vi "Intellirupter_basic.vi"() -> ()   [LabVIEW 2016]
uses:
  <vilib>/addons/Electrical Power/Protection/Definite Time Delay/subVIs/fpga_Time Delay Cfg.ctl
  <vilib>/FPGAPlugInAG/cRIO-9039 (Sync)/niLvFpga_Open_cRIO-9039 (Sync).vi
  <vilib>/rvi/interface/common/dynamic/niFpgaDynamicAddResources.vi
  <vilib>/Utility/error.llb/Error Cluster From Error Code.vi
  <vilib>/rvi/errors/niLvFpgaAdjustHostInterfaceError.vi
  <vilib>/FPGAPlugInAG/Dynamic/niLvFpga_Close_Dynamic.vi
  <vilib>/rvi/interface/nirviOpenFPGA/nirviOpenFPGA.xnode
  FPGA Bitfiles/IntelliRupter_calibrated.lvbitx
  <vilib>/rvi/interface/nirviReadWriteControl/nirviReadWriteControl.xnode
  <vilib>/rvi/interface/nirviCloseFPGA/nirviCloseFPGA.xnode
  <vilib>/rvi/interface/Simulation/niFpgaSimulationCallBeginRW.vi
  NiFpgaLv.dll
  <vilib>/addons/Electrical Power/Protection/NI_EP_Protection_FPGA.lvlib
panel:
  out "x-y":u32=48
  in  "Recloser Settings":T1={"Magnitude Minimum"=0.1, "Magnitude difference level"=0.005, "Frequency difference level"=0.5, "Phase difference level"=10.0}
  out "Trip Relay8":bool
  out "Trip Relay7":bool
  out "Trip Relay6":bool
  out "Trip Relay5":bool
  out "Trip Relay4":bool
  out "Trip Relay3":bool=TRUE
  out "Trip Relay2":bool
  out "Trip Relay1":bool
  out "MGCC_to_relay":bool[](array[boolean])=[TRUE, TRUE, FALSE, TRUE, TRUE, TRUE, TRUE, TRUE]
  out "Waveform Chart":dbl(graph)=-0.6613750457763672
  in  "Count(ticks)":u32=10000
  in  "RMS minimum\nvalues":T2={"VRMS values"=[0.5, 0.5, 0.5], "IRMS values"=[0.1, 0.1, 0.1]}
  out "error out":errorcluster
  out "Relay_toMGCC":bool[](array[boolean])=[TRUE, TRUE, FALSE, TRUE, TRUE, TRUE, TRUE, TRUE]
  in  "Manual trip Relay8":bool
  in  "Reclose Relay8?":bool=TRUE
  out "R8 Data for\ncommunication":dbl[](array[numeric])=[1.0, 0.9772472927114874, 0.9778624121532871, 61.827518463134766, 61.82509231567383, -3.8680694103240967, 0.13812482357025146, 0.006883656140416861, 0.0, 0.0]
  in  "Manual trip Relay7":bool
  in  "Reclose Relay7?":bool=TRUE
  out "R7 Data for\ncommunication":dbl[](array[numeric])=[1.0, 0.9791859731446678, 0.9754579902644022, 61.867767333984375, 61.880252838134766, -0.6613750457763672, -0.12970688939094543, -0.04306116700172424, 0.0, 0.0]
  in  "Manual trip Relay6":bool
  in  "Reclose Relay6?":bool=TRUE
  out "R6 Data for\ncommunication":dbl[](array[numeric])=[1.0, 0.9788151236253823, 0.9740843633835886, 61.9020881652832, 61.9046630859375, -2.975890874862671, 0.1713959127664566, 0.006507526151835918, 0.0, 0.0]
  in  "Manual trip Relay5":bool
  in  "Reclose Relay5?":bool=TRUE
  out "R5 Data for\ncommunication":dbl[](array[numeric])=[1.0, 0.9783700429887375, 0.9755752232502363, 61.90061569213867, 61.932212829589844, -2.8843889236450195, 0.1442330777645111, 0.0923943892121315, 0.0, 0.0]
  in  "Manual trip Relay4":bool
  in  "Reclose Relay4?":bool=TRUE
  out "R4 Data for\ncommunication":dbl[](array[numeric])=[1.0, 0.9780153533539752, 0.9771056813373646, 61.89913558959961, 61.91067123413086, 0.8295685648918152, 0.14155393838882446, 0.10946153849363327, 0.0, 0.0]
  in  "Manual trip Relay3":bool
  in  "Reclose Relay3?":bool
  out "R3 Data for\ncommunication":dbl[](array[numeric])=[0.0, 0.9772597508136373, 0.0028412240837732733, 61.94487380981445, 60.0, 87.80017852783203, 0.0009702712413854897, -0.00019450465333648026, 0.0, 0.0]
  in  "Manual trip Relay2":bool
  in  "Reclose Relay2?":bool=TRUE
  out "R2 Data for\ncommunication":dbl[](array[numeric])=[1.0, 0.9799129313520322, 0.9783522289749266, 61.984336853027344, 61.987144470214844, 4.425566673278809, 0.5318686962127686, 0.09335238486528397, 0.0, 0.0028076171875]
  out "R1 Data for\ncommunication":dbl[](array[numeric])=[1.0, 0.9830398860987186, 0.9848198490696459, 62.0186653137207, 62.001502990722656, 3.7592506408691406, 0.7891018986701965, 0.08714056760072708, 0.0, -0.017162322998046875]
  in  "Relay8":bool=TRUE
  in  "Relay7":bool=TRUE
  in  "Relay6":bool=TRUE
  in  "Relay5":bool=TRUE
  in  "Relay4":bool=TRUE
  in  "Relay3":bool
  in  "Relay2":bool=TRUE
  in  "Reclose Relay1?":bool=TRUE
  out "half cycle (samples)":i32=96
  out "basic calc interval":u16=2074
  in  "stop":bool
  in  "Relay1":bool=TRUE
  in  "Manual trip Relay1":bool
  # "status\nmag_left\nmag_right\nfreq_left\nfreq_right\nang_diff\nact_power\nrea_power\n0\n0"
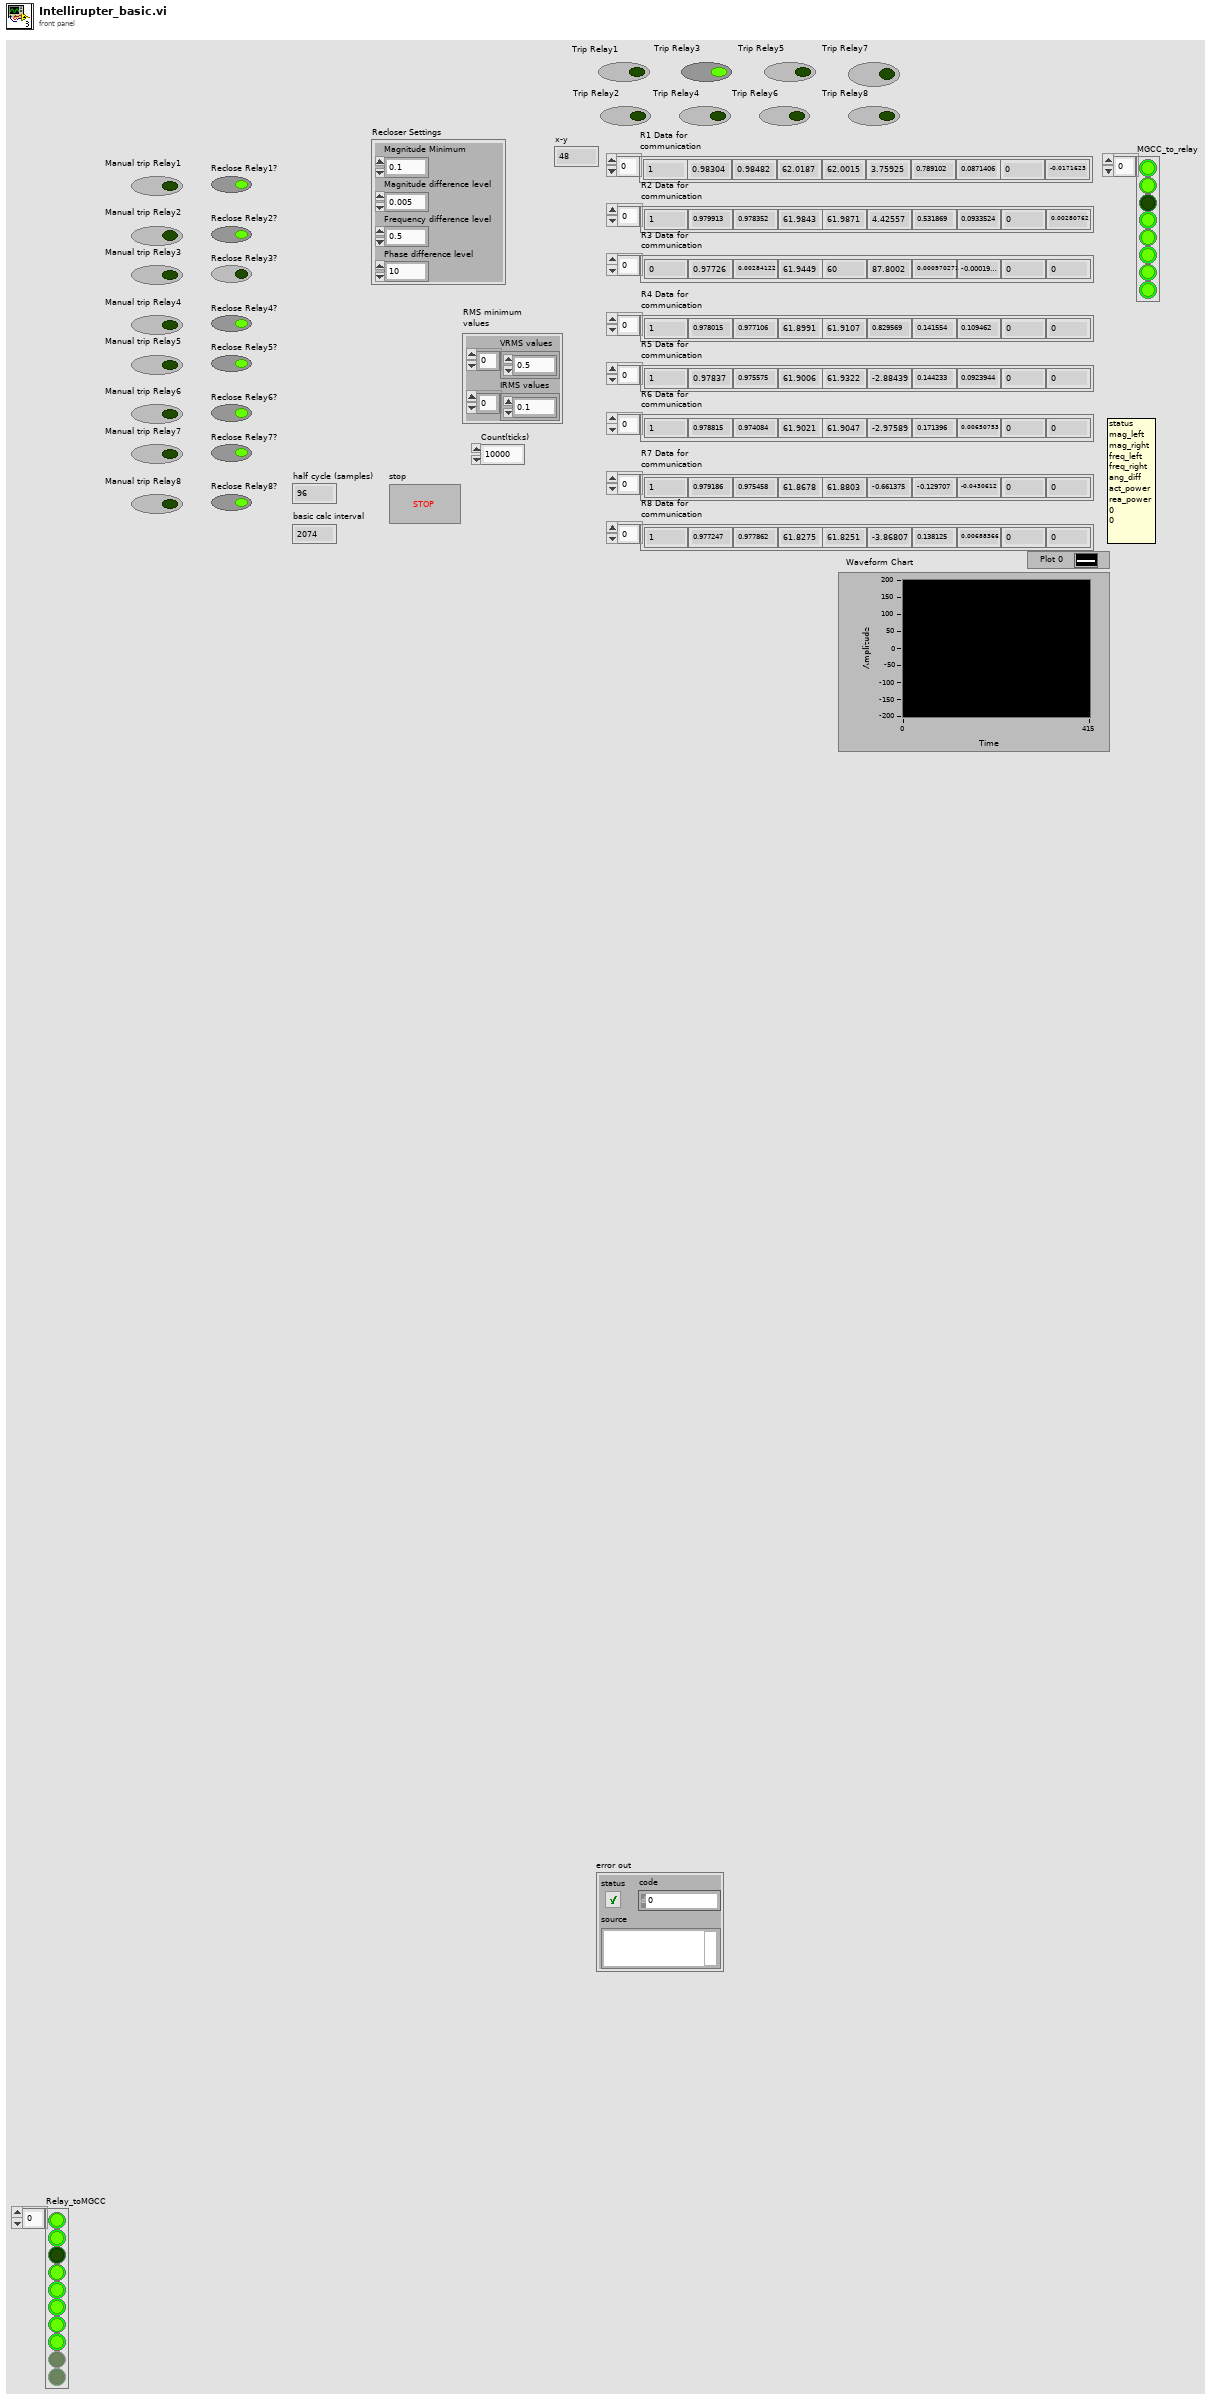
[diagram p1: front panel]
types:
  T1 = cluster{"Magnitude Minimum":dbl, "Magnitude difference level":dbl, "Frequency difference level":dbl, "Phase difference level":dbl}
  T2 = cluster{"VRMS values":dbl[], "IRMS values":dbl[]}
  T3 = cluster{fxp<+/-,53,11>[], fxp<+/-,53,11>[], fxp<+/-,53,11>[], fxp<+/-,53,11>[], fxp<+/-,53,11>[], fxp<+/-,53,11>[], fxp<+/-,53,11>[], fxp<+/-,53,11>[], fxp<+/-,53,11>[]}
  T4 = typedef "NI_EP_Protection_FPGA.lvlib/fpga_Time Delay Cfg.ctl" = cluster{"operate time [ms]":u32, "reset time [ms]":u32, "operate time compensation [ms]":u32}
  T5 = cluster{"UV Reset level":dbl, "Undervoltage \npick-up level":dbl, "OC Reset level":dbl, "Overcurrent\npick-up level":dbl, "time delay settings":T4}
  T6 = typedef "NI_EP_Protection_FPGA.lvlib/fpga_Timer Feedback Var.ctl" = cluster{"time elapsed":u32, "start time of trip counting":u32, "start time of reseting":u32}
  T7 = typedef "NI_EP_Protection_FPGA.lvlib/fpga_State.ctl" = enum16{"Idle", "Trip Counting", "Tripped", "Reset Counting"}
  T8 = cluster{bool, bool, "Boolean":bool, "timing values out":T6, "status out":T7, "trip signal out":bool}
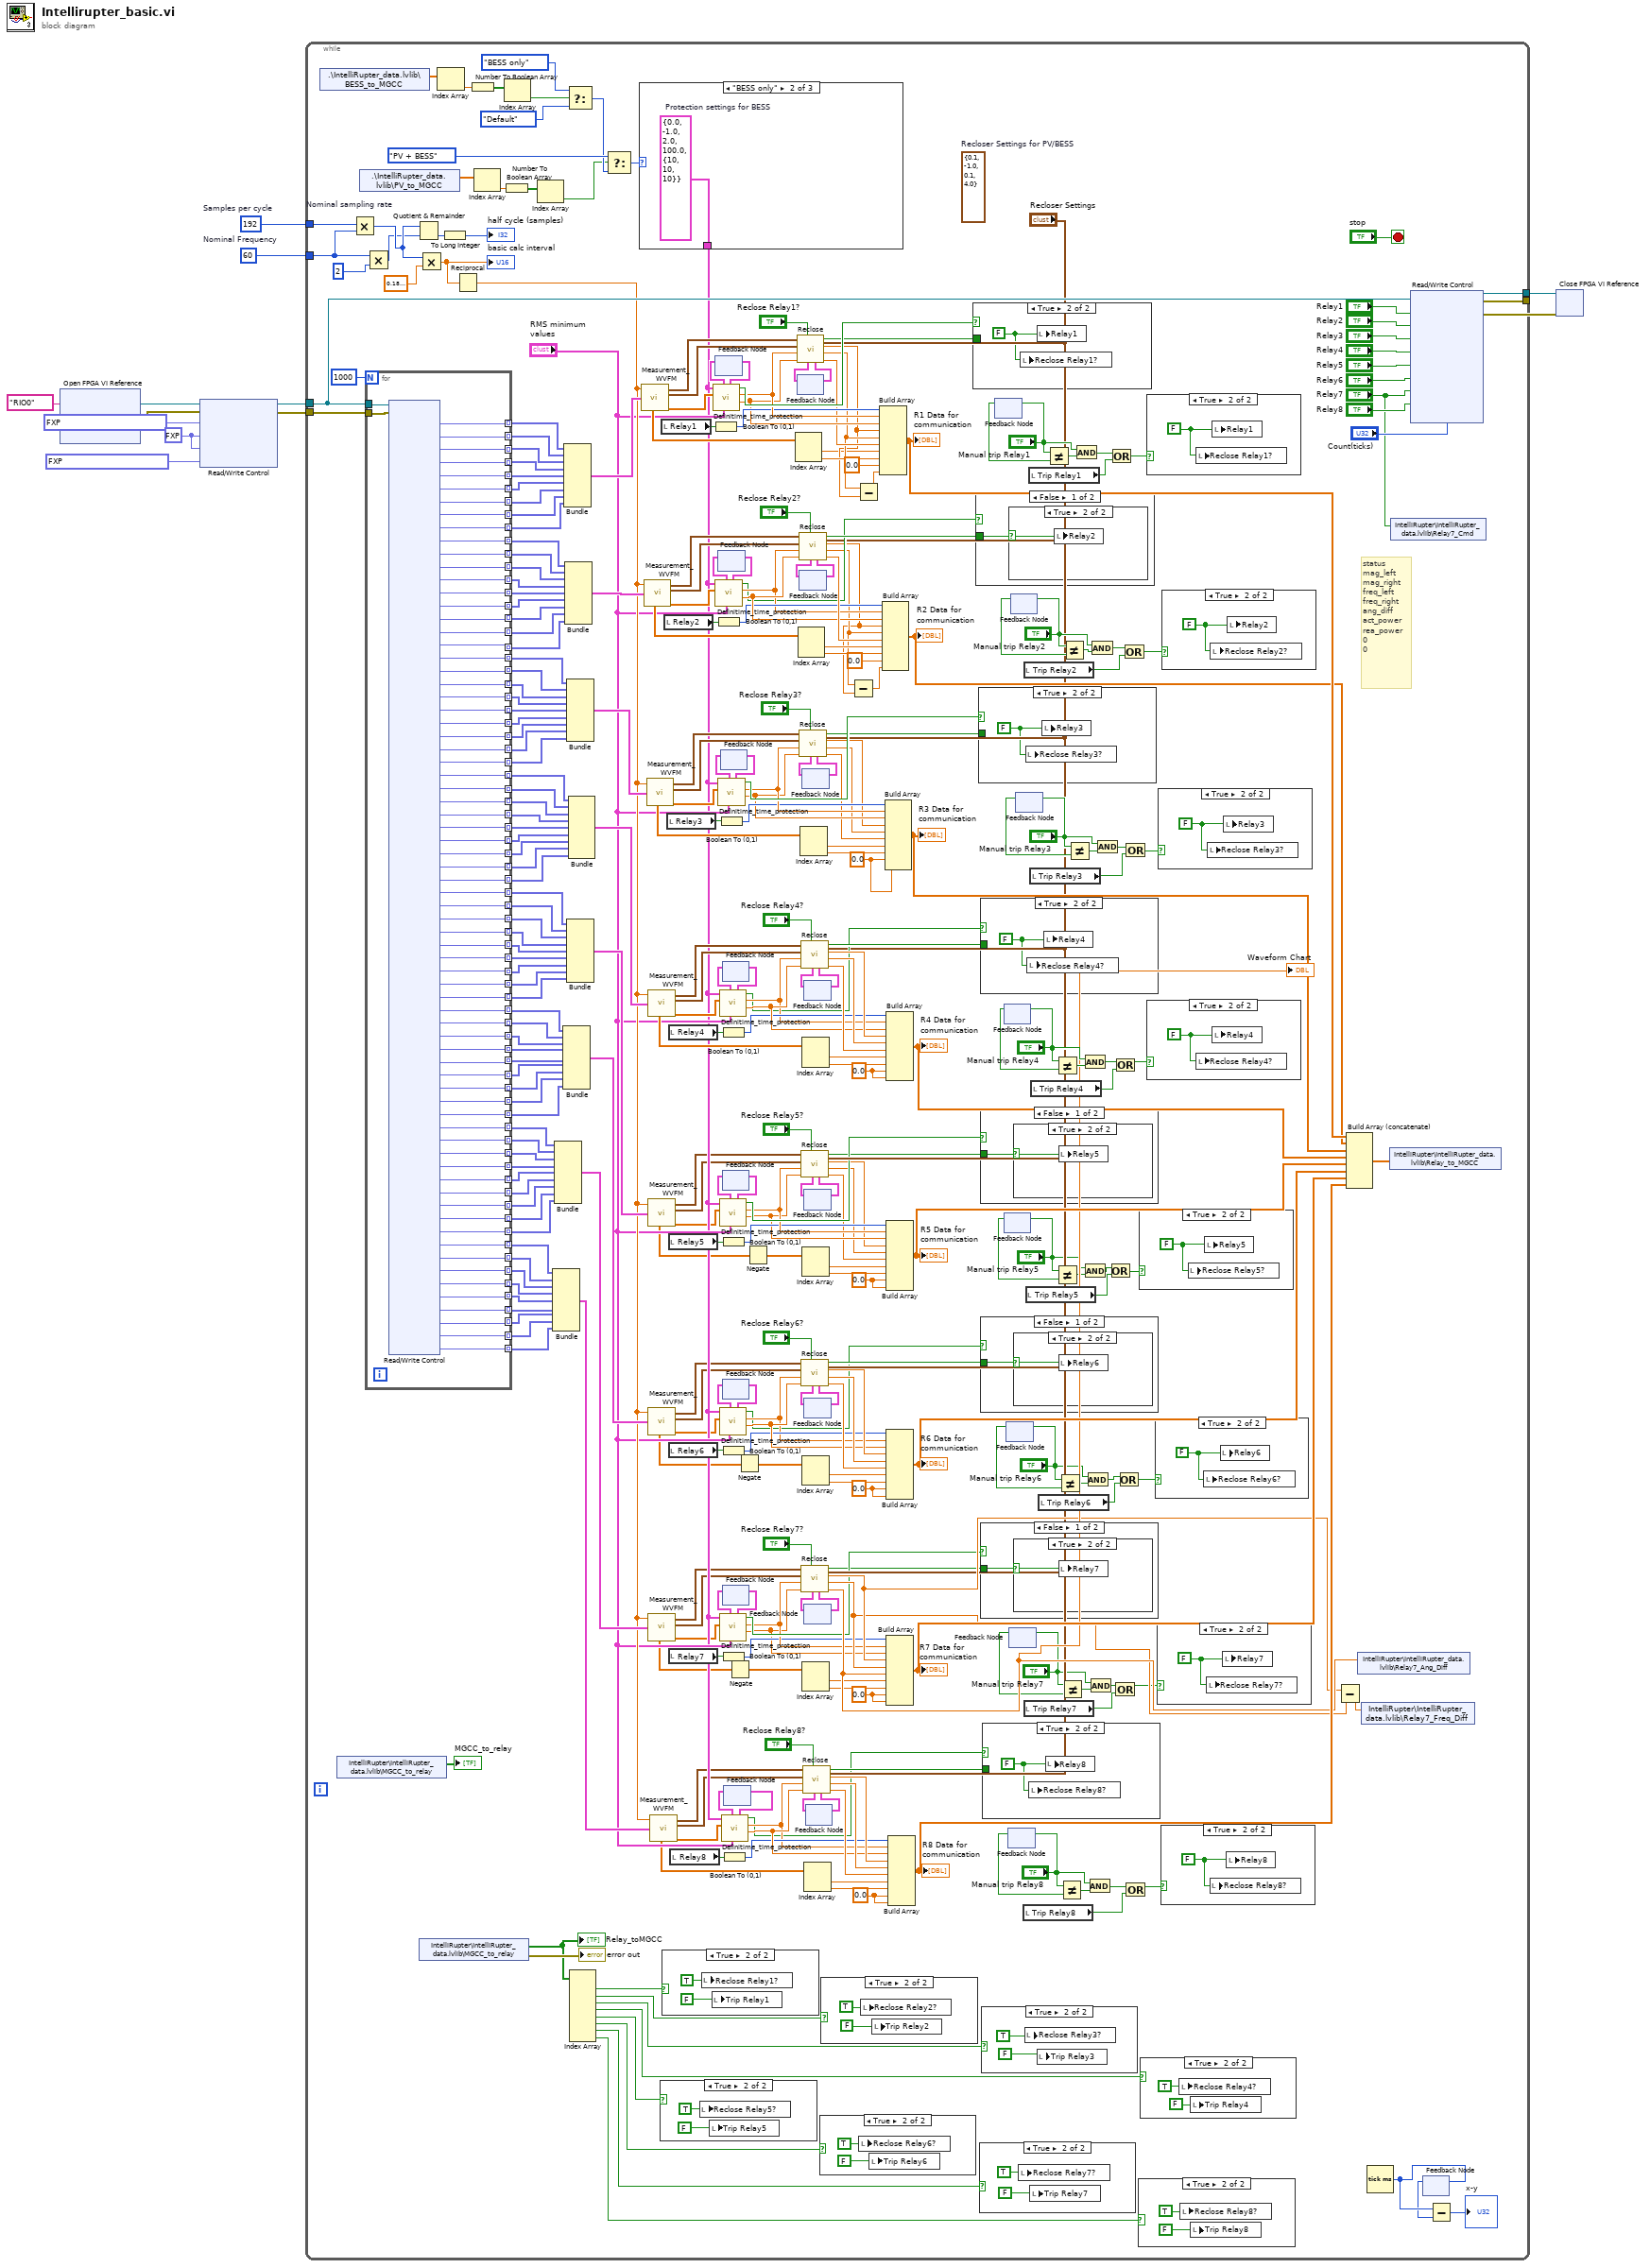
[diagram p0: block diagram]
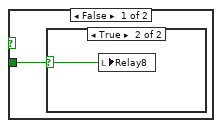
[diagram p2: hidden frame]
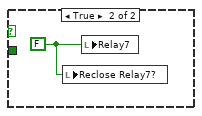
[diagram p6: hidden frame]
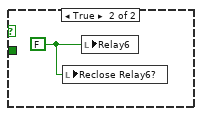
[diagram p9: hidden frame]
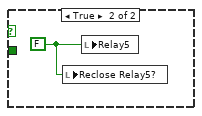
[diagram p12: hidden frame]
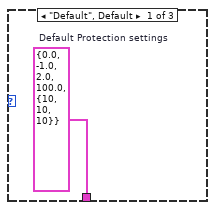
[diagram p14: hidden frame]
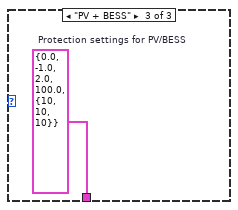
[diagram p15: hidden frame]
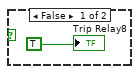
[diagram p16: hidden frame]
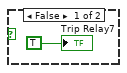
[diagram p17: hidden frame]
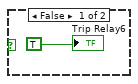
[diagram p18: hidden frame]
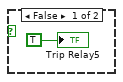
[diagram p19: hidden frame]
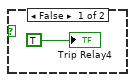
[diagram p20: hidden frame]
diagram:
  w2 = fxp<+/-,52,10> 0.0 ("I offset")
  w1 = 192  # Samples per cycle
  w10 = 60  # Nominal Frequency
  n1 = xnode "Open FPGA VI Reference"("resource name"=tag "RIO0") -> ("FPGA VI Reference Out"=w12:refnum<k20>, "error out"=w6:errorcluster)  [unwired: 1 in]
  n2 = xnode "Read/Write Control"("FPGA VI Reference In"=w12, "error in"=w6, "I scale factor"=fxp<+/-,26,5> 0.4850001335144043, "I offset"=w2, "V offset"=w2, "V scale factor"=fxp<+/-,26,5> 0.40000009536743164) -> ("FPGA VI Reference Out"=w7:refnum<k20>, "error out"=w5:errorcluster)
  n3 = while {
    tunnel: w7 -> [w363]
    tunnel: w10 -> [w371]
    tunnel: [w369] -> w9
    tunnel: [w368] -> w8
    tunnel: w5 -> [w362]
    tunnel: w1 -> [w176]
    stop <- "stop" stop-if-true
    w62 = 0.0 ("element")
    w63 = 0.0 ("element")
    w106 = 0.0 ("element")
    w107 = 0.0 ("element")
    (unwired) T1 {"Magnitude Minimum"=0.1, "Magnitude difference level"=-1.0, "Frequency difference level"=0.1, "Phase difference level"=4.0}  # Recloser Settings for PV/BESS
    w262 = 0.0 ("element")
    w272 = 0.0 ("element")
    # "status\nmag_left\nmag_right\nfreq_left\nfreq_right\nang_diff\nact_power\nrea_power\n0\n0"
    n4 = shared-variable ".\\IntelliRupter_data.lvlib\\BESS_to_MGCC"() -> (w134:dbl[])  [unwired: 1 in, 1 out]
    n5 = shared-variable "IntelliRupter\\IntelliRupter_data.lvlib\\MGCC_to_relay"() -> (→"MGCC_to_relay":bool[])  [unwired: 1 in, 1 out]
    n6 = Multiply "Nominal sampling rate"(x=w176, y=w371) -> (x*y=w377:i32)
    n7 = shared-variable ".\\IntelliRupter_data.lvlib\\PV_to_MGCC"() -> (w138:dbl[])  [unwired: 1 in, 1 out]
    n8 = Multiply(x=w371, y=2) -> (x*y=w373:i32)
    n9 = for {
      N: 1000 -> [_]
      tunnel: w363 -> [w507]
      tunnel: w362 -> [w506]
      tunnel: [w505] -> w360 mode=indexing
      tunnel: [w504] -> w359 mode=indexing
      tunnel: [w503] -> w358 mode=indexing
      tunnel: [w502] -> w357 mode=indexing
      tunnel: [w501] -> w356 mode=indexing
      tunnel: [w500] -> w355 mode=indexing
      tunnel: [w499] -> w354 mode=indexing
      tunnel: [w498] -> w353 mode=indexing
      tunnel: [w497] -> w352 mode=indexing
      tunnel: [w496] -> w326 mode=indexing
      tunnel: [w495] -> w325 mode=indexing
      tunnel: [w494] -> w324 mode=indexing
      tunnel: [w493] -> w323 mode=indexing
      tunnel: [w492] -> w322 mode=indexing
      tunnel: [w491] -> w321 mode=indexing
      tunnel: [w490] -> w320 mode=indexing
      tunnel: [w489] -> w319 mode=indexing
      tunnel: [w488] -> w318 mode=indexing
      tunnel: [w487] -> w271 mode=indexing
      tunnel: [w486] -> w270 mode=indexing
      tunnel: [w485] -> w269 mode=indexing
      tunnel: [w484] -> w268 mode=indexing
      tunnel: [w483] -> w267 mode=indexing
      tunnel: [w482] -> w266 mode=indexing
      tunnel: [w481] -> w265 mode=indexing
      tunnel: [w480] -> w264 mode=indexing
      tunnel: [w479] -> w263 mode=indexing
      tunnel: [w478] -> w237 mode=indexing
      tunnel: [w477] -> w236 mode=indexing
      tunnel: [w476] -> w235 mode=indexing
      tunnel: [w475] -> w234 mode=indexing
      tunnel: [w474] -> w233 mode=indexing
      tunnel: [w473] -> w232 mode=indexing
      tunnel: [w472] -> w231 mode=indexing
      tunnel: [w471] -> w230 mode=indexing
      tunnel: [w470] -> w229 mode=indexing
      tunnel: [w469] -> w228 mode=indexing
      tunnel: [w468] -> w227 mode=indexing
      tunnel: [w467] -> w226 mode=indexing
      tunnel: [w466] -> w225 mode=indexing
      tunnel: [w465] -> w224 mode=indexing
      tunnel: [w464] -> w223 mode=indexing
      tunnel: [w463] -> w222 mode=indexing
      tunnel: [w462] -> w221 mode=indexing
      tunnel: [w461] -> w220 mode=indexing
      tunnel: [w460] -> w218 mode=indexing
      tunnel: [w459] -> w217 mode=indexing
      tunnel: [w458] -> w216 mode=indexing
      tunnel: [w457] -> w215 mode=indexing
      tunnel: [w456] -> w214 mode=indexing
      tunnel: [w455] -> w213 mode=indexing
      tunnel: [w454] -> w212 mode=indexing
      tunnel: [w453] -> w211 mode=indexing
      tunnel: [w452] -> w210 mode=indexing
      tunnel: [w451] -> w208 mode=indexing
      tunnel: [w450] -> w207 mode=indexing
      tunnel: [w449] -> w206 mode=indexing
      tunnel: [w448] -> w205 mode=indexing
      tunnel: [w447] -> w204 mode=indexing
      tunnel: [w446] -> w203 mode=indexing
      tunnel: [w445] -> w202 mode=indexing
      tunnel: [w444] -> w201 mode=indexing
      tunnel: [w443] -> w200 mode=indexing
      tunnel: [w442] -> w198 mode=indexing
      tunnel: [w441] -> w197 mode=indexing
      tunnel: [w440] -> w196 mode=indexing
      tunnel: [w439] -> w195 mode=indexing
      tunnel: [w438] -> w194 mode=indexing
      tunnel: [w437] -> w193 mode=indexing
      tunnel: [w436] -> w192 mode=indexing
      tunnel: [w435] -> w191 mode=indexing
      tunnel: [w434] -> w190 mode=indexing
      n10 = xnode "Read/Write Control"("FPGA VI Reference In"=w507, "error in"=w506) -> ("V1L AB"=w505:fxp<+/-,53,11>, "V1L BC"=w504:fxp<+/-,53,11>, "V1L CA"=w503:fxp<+/-,53,11>, "V1R AB"=w502:fxp<+/-,53,11>, "V1R BC"=w501:fxp<+/-,53,11>, "V1R CA"=w500:fxp<+/-,53,11>, "I1 A"=w499:fxp<+/-,53,11>, "I1 B"=w498:fxp<+/-,53,11>, "I1 C"=w497:fxp<+/-,53,11>, "V2L AB"=w496:fxp<+/-,53,11>, "V2L BC"=w495:fxp<+/-,53,11>, "V2L CA"=w494:fxp<+/-,53,11>, "V2R AB"=w493:fxp<+/-,53,11>, "V2R BC"=w492:fxp<+/-,53,11>, "V2R CA"=w491:fxp<+/-,53,11>, "I2 A"=w490:fxp<+/-,53,11>, "I2 B"=w489:fxp<+/-,53,11>, "I2 C"=w488:fxp<+/-,53,11>, "V3L AB"=w487:fxp<+/-,53,11>, "V3L BC"=w486:fxp<+/-,53,11>, "V3L CA"=w485:fxp<+/-,53,11>, "V3R AB"=w484:fxp<+/-,53,11>, "V3R BC"=w483:fxp<+/-,53,11>, "V3R CA"=w482:fxp<+/-,53,11>, "I3 A"=w481:fxp<+/-,53,11>, "I3 B"=w480:fxp<+/-,53,11>, "I3 C"=w479:fxp<+/-,53,11>, "V4L AB"=w478:fxp<+/-,53,11>, "V4L BC"=w477:fxp<+/-,53,11>, "V4L CA"=w476:fxp<+/-,53,11>, "V4R AB"=w475:fxp<+/-,53,11>, "V4R BC"=w474:fxp<+/-,53,11>, "V4R CA"=w473:fxp<+/-,53,11>, "I4 A"=w472:fxp<+/-,53,11>, "I4 B"=w471:fxp<+/-,53,11>, "I4 C"=w470:fxp<+/-,53,11>, "V5L AB"=w469:fxp<+/-,53,11>, "V5L BC"=w468:fxp<+/-,53,11>, "V5L CA"=w467:fxp<+/-,53,11>, "V5R AB"=w466:fxp<+/-,53,11>, "V5R BC"=w465:fxp<+/-,53,11>, "V5R CA"=w464:fxp<+/-,53,11>, "I5 A"=w463:fxp<+/-,53,11>, "I5 B"=w462:fxp<+/-,53,11>, "I5 C"=w461:fxp<+/-,53,11>, "V6L AB"=w460:fxp<+/-,53,11>, "V6L BC"=w459:fxp<+/-,53,11>, "V6L CA"=w458:fxp<+/-,53,11>, "V6R AB"=w457:fxp<+/-,53,11>, "V6R BC"=w456:fxp<+/-,53,11>, "V6R CA"=w455:fxp<+/-,53,11>, "I6 A"=w454:fxp<+/-,53,11>, "I6 B"=w453:fxp<+/-,53,11>, "I6 C"=w452:fxp<+/-,53,11>, "V7L AB"=w451:fxp<+/-,53,11>, "V7L BC"=w450:fxp<+/-,53,11>, "V7L CA"=w449:fxp<+/-,53,11>, "V7R AB"=w448:fxp<+/-,53,11>, "V7R BC"=w447:fxp<+/-,53,11>, "V7R CA"=w446:fxp<+/-,53,11>, "I7 A"=w445:fxp<+/-,53,11>, "I7 B"=w444:fxp<+/-,53,11>, "I7 C"=w443:fxp<+/-,53,11>, "V8L AB"=w442:fxp<+/-,53,11>, "V8L BC"=w441:fxp<+/-,53,11>, "V8L CA"=w440:fxp<+/-,53,11>, "V8R AB"=w439:fxp<+/-,53,11>, "V8R BC"=w438:fxp<+/-,53,11>, "V8R CA"=w437:fxp<+/-,53,11>, "I8 A"=w436:fxp<+/-,53,11>, "I8 B"=w435:fxp<+/-,53,11>, "I8 C"=w434:fxp<+/-,53,11>)  [unwired: 2 out]
    }
    n11 = Quotient & Remainder(x=w377, y=w373) -> (floor(x/y)=w375:i32)  [unwired: 1 out]
    n12 = Multiply(x=w377, y=sgl 0.18) -> (x*y=w378:sgl)
    "basic calc interval" <- w378
    n13 = shared-variable "IntelliRupter\\IntelliRupter_data.lvlib\\MGCC_to_relay"() -> (w172:bool[], error out=→"error out":errorcluster)  [unwired: 1 in]
    "Relay_toMGCC" <- w172
    n14 = Index Array(array=w134) -> (element=w133:dbl)  [unwired: 1 in]
    n15 = To Long Integer(number=w375) -> (32bit integer=→"half cycle (samples)":i32)
    n16 = Reciprocal(x=w378) -> (1/x=w189:sgl)
    n17 = Number To Boolean Array(number=w133) -> (Boolean array=w142:bool[])
    n18 = Index Array(array=w138) -> (element=w137:dbl)  [unwired: 1 in]
    n19 = Number To Boolean Array(number=w137) -> (Boolean array=w136:bool[])
    n20 = Index Array(array=w142) -> (element=w141:bool)  [unwired: 1 in]
    n21 = Index Array(array=w136) -> (element=w135:bool)  [unwired: 1 in]
    n22 = Bundle(w198, w197, w196, w195, w194, w193, w192, w191, w190) -> (w188:T3)  [unwired: 1 in]
    n23 = Bundle(w208, w207, w206, w205, w204, w203, w202, w201, w200) -> (w199:T3)  [unwired: 1 in]
    n24 = Bundle(w218, w217, w216, w215, w214, w213, w212, w211, w210) -> (w209:T3)  [unwired: 1 in]
    n25 = Bundle(w360, w359, w358, w357, w356, w355, w354, w353, w352) -> (w351:T3)  [unwired: 1 in]
    n26 = Bundle(w326, w325, w324, w323, w322, w321, w320, w319, w318) -> (w296:T3)  [unwired: 1 in]
    n27 = Select(t=enum16{"Default", "BESS only", "PV + BESS"}."BESS only", s=w141, f=enum16{"Default", "BESS only", "PV + BESS"}."Default") -> (s? t:f=w143:enum16{"Default", "BESS only", "PV + BESS"})
    n28 = Bundle(w271, w270, w269, w268, w267, w266, w265, w264, w263) -> (w295:T3)  [unwired: 1 in]
    n29 = Bundle(w228, w227, w226, w225, w224, w223, w222, w221, w220) -> (w219:T3)  [unwired: 1 in]
    n30 = Bundle(w237, w236, w235, w234, w233, w232, w231, w230, w229) -> (w238:T3)  [unwired: 1 in]
    n31 = Index Array(array=w172) -> (element #1=w171:bool, element #2=w170:bool, element #3=w169:bool, element #4=w168:bool, element #5=w167:bool, element #6=w166:bool, element #7=w165:bool, element #8=w164:bool)  [unwired: 8 in]
    n32 = Select(t=enum16{"Default", "BESS only", "PV + BESS"}."PV + BESS", s=w135, f=w143) -> (s? t:f=w145:enum16{"Default", "BESS only", "PV + BESS"})
    n33 = case shown="\"BESS only\"" w145 {
      tunnel: [w395 w396 w397] -> w146
      frame "Default", Default {
        w395 = T5 {"UV Reset level"=0.0, "Undervoltage \npick-up level"=-1.0, "OC Reset level"=2.0, "Overcurrent\npick-up level"=100.0, "time delay settings"={"operate time [ms]"=10, "reset time [ms]"=10, "operate time compensation [ms]"=10}}  # Default Protection settings
      }
      frame "BESS only" {
        w396 = T5 {"UV Reset level"=0.0, "Undervoltage \npick-up level"=-1.0, "OC Reset level"=2.0, "Overcurrent\npick-up level"=100.0, "time delay settings"={"operate time [ms]"=10, "reset time [ms]"=10, "operate time compensation [ms]"=10}}  # Protection settings for BESS
      }
      frame "PV + BESS" {
        w397 = T5 {"UV Reset level"=0.0, "Undervoltage \npick-up level"=-1.0, "OC Reset level"=2.0, "Overcurrent\npick-up level"=100.0, "time delay settings"={"operate time [ms]"=10, "reset time [ms]"=10, "operate time compensation [ms]"=10}}  # Protection settings for PV/BESS
      }
    }
    n34 = call "Measurement_WVFM.vi"("dt"=w189, "Input cluster"=w351) -> ("Total power values"=w335:dbl[], "VL array"=w350:waveform(sgl)[], "VR array"=w349:waveform(sgl)[], "Active Power"=w155:dbl[])  [unwired: 2 in, 1 out]
    n35 = call "Measurement_WVFM.vi"("dt"=w189, "Input cluster"=w296) -> ("Total power values"=w315:dbl[], "VL array"=w301:waveform(sgl)[], "VR array"=w302:waveform(sgl)[], "Active Power"=w154:dbl[])  [unwired: 2 in, 1 out]
    n36 = call "Measurement_WVFM.vi"("dt"=w189, "Input cluster"=w295) -> ("Total power values"=w274:dbl[], "VL array"=w290:waveform(sgl)[], "VR array"=w289:waveform(sgl)[], "Active Power"=w153:dbl[])  [unwired: 2 in, 1 out]
    n37 = call "Measurement_WVFM.vi"("dt"=w189, "Input cluster"=w238) -> ("Total power values"=w259:dbl[], "VL array"=w243:waveform(sgl)[], "VR array"=w244:waveform(sgl)[], "Active Power"=w152:dbl[])  [unwired: 2 in, 1 out]
    n38 = call "Measurement_WVFM.vi"("dt"=w189, "Input cluster"=w219) -> ("Total power values"=w110:dbl[], "VL array"=w126:waveform(sgl)[], "VR array"=w125:waveform(sgl)[], "Active Power"=w29:dbl[])  [unwired: 2 in, 1 out]
    n39 = call "Measurement_WVFM.vi"("dt"=w189, "Input cluster"=w209) -> ("Total power values"=w83:dbl[], "VL array"=w88:waveform(sgl)[], "VR array"=w89:waveform(sgl)[], "Active Power"=w28:dbl[])  [unwired: 2 in, 1 out]
    n40 = call "Measurement_WVFM.vi"("dt"=w189, "Input cluster"=w199) -> ("Total power values"=w82:dbl[], "VL array"=w77:waveform(sgl)[], "VR array"=w76:waveform(sgl)[], "Active Power"=w27:dbl[])  [unwired: 2 in, 1 out]
    n41 = call "Measurement_WVFM.vi"("dt"=w189, "Input cluster"=w188) -> ("Total power values"=w39:dbl[], "VL array"=w44:waveform(sgl)[], "VR array"=w45:waveform(sgl)[], "Active Power"=w26:dbl[])  [unwired: 2 in, 1 out]
    n42 = case shown="True" w167 {
      frame False {
        "Trip Relay5" <- TRUE ("Manual trip Relay1")
      }
      frame True {
        n43 = local write "Reclose Relay5?"(TRUE ("Reclose Relay1?")) -> ()
        n44 = local write "Trip Relay5"(FALSE ("Reclose Relay1?")) -> ()
      }
    }
    n45 = local read "Relay1"() -> (w340:bool)
    n46 = case shown="True" w171 {
      frame False {
        "Trip Relay1" <- TRUE ("Manual trip Relay1")
      }
      frame True {
        n47 = local write "Reclose Relay1?"(TRUE ("Reclose Relay1?")) -> ()
        n48 = local write "Trip Relay1"(FALSE ("Reclose Relay1?")) -> ()
      }
    }
    n49 = local read "Relay2"() -> (w310:bool)
    n50 = local read "Relay3"() -> (w281:bool)
    n51 = local read "Relay4"() -> (w252:bool)
    n52 = local read "Relay5"() -> (w117:bool)
    n53 = local read "Relay6"() -> (w97:bool)
    n54 = local read "Relay7"() -> (w68:bool)
    n55 = local read "Relay8"() -> (w53:bool)
    n56 = Boolean To (0,1)(Boolean=w340) -> (0, 1=w338:i16)
    n57 = feedback #1() -> (w347:T8)  [unwired: 1 in]
    n58 = call "Definitime_time_protection.vi"("RMS minimum\nvalues"="RMS minimum\nvalues", "input cluster"=w347, "Active Power"=w155, "Protection settings"=w146) -> ("VR RMS"=w337:dbl, "VL RMS"=w339:dbl, "trip signal"=w343:bool, "output cluster"=w348:T8)  [unwired: 2 in, 2 out]
    n59 = feedback-in #1(w348) -> ()
    n60 = Boolean To (0,1)(Boolean=w310) -> (0, 1=w312:i16)
    n61 = feedback #2() -> (w304:T8)  [unwired: 1 in]
    n62 = call "Definitime_time_protection.vi"("RMS minimum\nvalues"="RMS minimum\nvalues", "input cluster"=w304, "Active Power"=w154, "Protection settings"=w146) -> ("VR RMS"=w313:dbl, "VL RMS"=w311:dbl, "trip signal"=w308:bool, "output cluster"=w303:T8)  [unwired: 2 in, 2 out]
    n63 = feedback-in #2(w303) -> ()
    n64 = Boolean To (0,1)(Boolean=w281) -> (0, 1=w279:i16)
    n65 = Boolean To (0,1)(Boolean=w252) -> (0, 1=w254:i16)
    n66 = Boolean To (0,1)(Boolean=w117) -> (0, 1=w115:i16)
    n67 = Boolean To (0,1)(Boolean=w97) -> (0, 1=w99:i16)
    n68 = Boolean To (0,1)(Boolean=w68) -> (0, 1=w66:i16)
    n69 = feedback #3() -> (w287:T8)  [unwired: 1 in]
    n70 = call "Definitime_time_protection.vi"("RMS minimum\nvalues"="RMS minimum\nvalues", "input cluster"=w287, "Active Power"=w153, "Protection settings"=w146) -> ("VR RMS"=w278:dbl, "VL RMS"=w280:dbl, "trip signal"=w283:bool, "output cluster"=w288:T8)  [unwired: 2 in, 2 out]
    n71 = feedback-in #3(w288) -> ()
    n72 = Boolean To (0,1)(Boolean=w53) -> (0, 1=w55:i16)
    n73 = feedback #4() -> (w246:T8)  [unwired: 1 in]
    n74 = call "Definitime_time_protection.vi"("RMS minimum\nvalues"="RMS minimum\nvalues", "input cluster"=w246, "Active Power"=w152, "Protection settings"=w146) -> ("VR RMS"=w255:dbl, "VL RMS"=w253:dbl, "trip signal"=w250:bool, "output cluster"=w245:T8)  [unwired: 2 in, 2 out]
    n75 = feedback-in #4(w245) -> ()
    n76 = feedback #5() -> (w123:T8)  [unwired: 1 in]
    n77 = call "Definitime_time_protection.vi"("RMS minimum\nvalues"="RMS minimum\nvalues", "input cluster"=w123, "Active Power"=w29, "Protection settings"=w146) -> ("VR RMS"=w114:dbl, "VL RMS"=w116:dbl, "trip signal"=w119:bool, "output cluster"=w124:T8)  [unwired: 2 in, 2 out]
    n78 = feedback-in #5(w124) -> ()
    n79 = feedback #6() -> (w91:T8)  [unwired: 1 in]
    n80 = call "Definitime_time_protection.vi"("RMS minimum\nvalues"="RMS minimum\nvalues", "input cluster"=w91, "Active Power"=w28, "Protection settings"=w146) -> ("VR RMS"=w100:dbl, "VL RMS"=w98:dbl, "trip signal"=w95:bool, "output cluster"=w90:T8)  [unwired: 2 in, 2 out]
    n81 = feedback-in #6(w90) -> ()
    n82 = feedback #7() -> (w74:T8)  [unwired: 1 in]
    n83 = call "Definitime_time_protection.vi"("RMS minimum\nvalues"="RMS minimum\nvalues", "input cluster"=w74, "Active Power"=w27, "Protection settings"=w146) -> ("VR RMS"=w65:dbl, "VL RMS"=w67:dbl, "trip signal"=w70:bool, "output cluster"=w75:T8)  [unwired: 2 in, 2 out]
    n84 = feedback-in #7(w75) -> ()
    n85 = feedback #8() -> (w47:T8)  [unwired: 1 in]
    n86 = call "Definitime_time_protection.vi"("RMS minimum\nvalues"="RMS minimum\nvalues", "input cluster"=w47, "Active Power"=w26, "Protection settings"=w146) -> ("VR RMS"=w56:dbl, "VL RMS"=w54:dbl, "trip signal"=w51:bool, "output cluster"=w46:T8)  [unwired: 2 in, 2 out]
    n87 = feedback-in #8(w46) -> ()
    n88 = Negate(x=w82) -> (-x=w25:dbl[])
    n89 = Negate(x=w83) -> (-x=w24:dbl[])
    n90 = Negate(x=w110) -> (-x=w23:dbl[])
    n91 = Index Array(array=w335) -> (element #1=w13:dbl, element #2=w334:dbl)  [unwired: 2 in]
    n92 = feedback #9() -> (w345:cluster{bool, dbl})  [unwired: 1 in]
    n93 = call "Reclose.vi"("Recloser Settings"="Recloser Settings", "Recloser in"=w345, "Reclose?"="Reclose Relay1?", "VR RMS avg"=w337, "VL RMS avg"=w339, "VR array"=w349, "VL array"=w350) -> ("Phase difference"=w336:dbl, "VR Frequency"=w21:dbl, "VL Frequency"=w20:dbl, "Recloser action"=w342:bool, "Recloser out"=w346:cluster{bool, dbl})
    n94 = feedback-in #9(w346) -> ()
    n95 = Index Array(array=w315) -> (element #1=w316:dbl, element #2=w317:dbl)  [unwired: 2 in]
    n96 = feedback #10() -> (w306:cluster{bool, dbl})  [unwired: 1 in]
    n97 = call "Reclose.vi"("Recloser Settings"="Recloser Settings", "Recloser in"=w306, "Reclose?"="Reclose Relay2?", "VR RMS avg"=w313, "VL RMS avg"=w311, "VR array"=w302, "VL array"=w301) -> ("Phase difference"=w314:dbl, "VR Frequency"=w17:dbl, "VL Frequency"=w16:dbl, "Recloser action"=w309:bool, "Recloser out"=w305:cluster{bool, dbl})
    n98 = feedback-in #10(w305) -> ()
    n99 = Index Array(array=w274) -> (element #1=w175:dbl, element #2=w273:dbl)  [unwired: 2 in]
    n100 = feedback #11() -> (w285:cluster{bool, dbl})  [unwired: 1 in]
    n101 = call "Reclose.vi"("Recloser Settings"="Recloser Settings", "Recloser in"=w285, "Reclose?"="Reclose Relay3?", "VR RMS avg"=w278, "VL RMS avg"=w280, "VR array"=w289, "VL array"=w290) -> ("Phase difference"=w275:dbl, "VR Frequency"=w276:dbl, "VL Frequency"=w277:dbl, "Recloser action"=w282:bool, "Recloser out"=w286:cluster{bool, dbl})
    n102 = feedback-in #11(w286) -> ()
    n103 = Index Array(array=w259) -> (element #1=w260:dbl, element #2=w261:dbl)  [unwired: 2 in]
    n104 = Index Array(array=w23) -> (element #1=w109:dbl, element #2=w108:dbl)  [unwired: 2 in]
    n105 = Index Array(array=w24) -> (element #1=w104:dbl, element #2=w105:dbl)  [unwired: 2 in]
    n106 = Index Array(array=w25) -> (element #1=w38:dbl, element #2=w64:dbl)  [unwired: 2 in]
    n107 = feedback #12() -> (w248:cluster{bool, dbl})  [unwired: 1 in]
    n108 = call "Reclose.vi"("Recloser Settings"="Recloser Settings", "Recloser in"=w248, "Reclose?"="Reclose Relay4?", "VR RMS avg"=w255, "VL RMS avg"=w253, "VR array"=w244, "VL array"=w243) -> ("Phase difference"=w258:dbl, "VR Frequency"=w257:dbl, "VL Frequency"=w256:dbl, "Recloser action"=w251:bool, "Recloser out"=w247:cluster{bool, dbl})
    n109 = feedback-in #12(w247) -> ()
    n110 = feedback #13() -> (w121:cluster{bool, dbl})  [unwired: 1 in]
    n111 = call "Reclose.vi"("Recloser Settings"="Recloser Settings", "Recloser in"=w121, "Reclose?"="Reclose Relay5?", "VR RMS avg"=w114, "VL RMS avg"=w116, "VR array"=w125, "VL array"=w126) -> ("Phase difference"=w111:dbl, "VR Frequency"=w112:dbl, "VL Frequency"=w113:dbl, "Recloser action"=w118:bool, "Recloser out"=w122:cluster{bool, dbl})
    n112 = feedback-in #13(w122) -> ()
    n113 = feedback #14() -> (w93:cluster{bool, dbl})  [unwired: 1 in]
    n114 = call "Reclose.vi"("Recloser Settings"="Recloser Settings", "Recloser in"=w93, "Reclose?"="Reclose Relay6?", "VR RMS avg"=w100, "VL RMS avg"=w98, "VR array"=w89, "VL array"=w88) -> ("Phase difference"=w103:dbl, "VR Frequency"=w102:dbl, "VL Frequency"=w101:dbl, "Recloser action"=w96:bool, "Recloser out"=w92:cluster{bool, dbl})
    n115 = feedback-in #14(w92) -> ()
    n116 = feedback #15() -> (w72:cluster{bool, dbl})  [unwired: 1 in]
    n117 = call "Reclose.vi"("Recloser Settings"="Recloser Settings", "Recloser in"=w72, "Reclose?"="Reclose Relay7?", "VR RMS avg"=w65, "VL RMS avg"=w67, "VR array"=w76, "VL array"=w77) -> ("Phase difference"=w151:dbl, "VR Frequency"=w149:dbl, "VL Frequency"=w150:dbl, "Recloser action"=w69:bool, "Recloser out"=w73:cluster{bool, dbl})
    "Waveform Chart" <- w151
    n118 = feedback-in #15(w73) -> ()
    n119 = Index Array(array=w39) -> (element #1=w60:dbl, element #2=w61:dbl)  [unwired: 2 in]
    n120 = feedback #16() -> (w49:cluster{bool, dbl})  [unwired: 1 in]
    n121 = call "Reclose.vi"("Recloser Settings"="Recloser Settings", "Recloser in"=w49, "Reclose?"="Reclose Relay8?", "VR RMS avg"=w56, "VL RMS avg"=w54, "VR array"=w45, "VL array"=w44) -> ("Phase difference"=w59:dbl, "VR Frequency"=w58:dbl, "VL Frequency"=w57:dbl, "Recloser action"=w52:bool, "Recloser out"=w48:cluster{bool, dbl})
    n122 = feedback-in #16(w48) -> ()
    n123 = case shown="True" w166 {
      frame False {
        "Trip Relay6" <- TRUE ("Manual trip Relay1")
      }
      frame True {
        n124 = local write "Reclose Relay6?"(TRUE ("Reclose Relay1?")) -> ()
        n125 = local write "Trip Relay6"(FALSE ("Reclose Relay1?")) -> ()
      }
    }
    n126 = case shown="True" w170 {
      frame False {
        "Trip Relay2" <- TRUE ("Manual trip Relay1")
      }
      frame True {
        n127 = local write "Reclose Relay2?"(TRUE ("Reclose Relay1?")) -> ()
        n128 = local write "Trip Relay2"(FALSE ("Reclose Relay1?")) -> ()
      }
    }
    n129 = Subtract(x=w17, y=w16) -> (x-y=w18:dbl)
    n130 = Subtract(x=w21, y=w20) -> (x-y=w22:dbl)
    n131 = Build Array(w338, w339, w337, w20, w21, w336, w13, w334, 0.0 ("element"), w22) -> (w186:dbl[])
    "R1 Data for\ncommunication" <- w186
    n132 = Build Array(w312, w311, w313, w16, w17, w314, w316, w317, 0.0 ("element"), w18) -> (w185:dbl[])
    "R2 Data for\ncommunication" <- w185
    n133 = Build Array(w279, w280, w278, w277, w276, w275, w175, w273, w272, w272) -> (w184:dbl[])
    "R3 Data for\ncommunication" <- w184
    n134 = Build Array(w254, w253, w255, w256, w257, w258, w260, w261, w262, w262) -> (w183:dbl[])
    "R4 Data for\ncommunication" <- w183
    n135 = Build Array(w115, w116, w114, w113, w112, w111, w109, w108, w107, w107) -> (w182:dbl[])
    "R5 Data for\ncommunication" <- w182
    n136 = Build Array(w99, w98, w100, w101, w102, w103, w104, w105, w106, w106) -> (w181:dbl[])
    "R6 Data for\ncommunication" <- w181
    n137 = Build Array(w66, w67, w65, w150, w149, w151, w38, w64, w63, w63) -> (w180:dbl[])
    "R7 Data for\ncommunication" <- w180
    n138 = Build Array(w55, w54, w56, w57, w58, w59, w60, w61, w62, w62) -> (w179:dbl[])
    "R8 Data for\ncommunication" <- w179
    n139 = case shown="True" w343 {
      tunnel: w342 -> [w508 _]
      frame False {
        n140 = case shown="True" w508 {
          selector: w508 -> [_ w509]
          frame False {
          }
          frame True {
            n141 = local write "Relay1"(w509) -> ()
          }
        }
      }
      frame True {
        w510 = FALSE ("Relay7")
        n142 = local write "Reclose Relay1?"(w510) -> ()
        n143 = local write "Relay1"(w510) -> ()
      }
    }
    n144 = case shown="False" w308 {
      tunnel: w309 -> [w430 _]
      frame False {
        n145 = case shown="True" w430 {
          selector: w430 -> [_ w431]
          frame False {
          }
          frame True {
            n146 = local write "Relay2"(w431) -> ()
          }
        }
      }
      frame True {
        w432 = FALSE ("Relay7")
        n147 = local write "Reclose Relay2?"(w432) -> ()
        n148 = local write "Relay2"(w432) -> ()
      }
    }
    n149 = case shown="True" w283 {
      tunnel: w282 -> [w426 _]
      frame False {
        n150 = case shown="True" w426 {
          selector: w426 -> [_ w427]
          frame False {
          }
          frame True {
            n151 = local write "Relay3"(w427) -> ()
          }
        }
      }
      frame True {
        w428 = FALSE ("Relay7")
        n152 = local write "Reclose Relay3?"(w428) -> ()
        n153 = local write "Relay3"(w428) -> ()
      }
    }
    n154 = case shown="True" w165 {
      frame False {
        "Trip Relay7" <- TRUE ("Manual trip Relay1")
      }
      frame True {
        n155 = local write "Reclose Relay7?"(TRUE ("Reclose Relay1?")) -> ()
        n156 = local write "Trip Relay7"(FALSE ("Reclose Relay1?")) -> ()
      }
    }
    n157 = case shown="True" w250 {
      tunnel: w251 -> [w422 _]
      frame False {
        n158 = case shown="True" w422 {
          selector: w422 -> [_ w423]
          frame False {
          }
          frame True {
            n159 = local write "Relay4"(w423) -> ()
          }
        }
      }
      frame True {
        w424 = FALSE ("Relay7")
        n160 = local write "Reclose Relay4?"(w424) -> ()
        n161 = local write "Relay4"(w424) -> ()
      }
    }
    n162 = case shown="False" w119 {
      tunnel: w118 -> [w391 _]
      frame False {
        n163 = case shown="True" w391 {
          selector: w391 -> [_ w392]
          frame False {
          }
          frame True {
            n164 = local write "Relay5"(w392) -> ()
          }
        }
      }
      frame True {
        w393 = FALSE ("Relay7")
        n165 = local write "Reclose Relay5?"(w393) -> ()
        n166 = local write "Relay5"(w393) -> ()
      }
    }
    n167 = case shown="False" w95 {
      tunnel: w96 -> [w387 _]
      frame False {
        n168 = case shown="True" w387 {
          selector: w387 -> [_ w388]
          frame False {
          }
          frame True {
            n169 = local write "Relay6"(w388) -> ()
          }
        }
      }
      frame True {
        w389 = FALSE ("Relay7")
        n170 = local write "Reclose Relay6?"(w389) -> ()
        n171 = local write "Relay6"(w389) -> ()
      }
    }
    n172 = case shown="False" w70 {
      tunnel: w69 -> [w383 _]
      frame False {
        n173 = case shown="True" w383 {
          selector: w383 -> [_ w384]
          frame False {
          }
          frame True {
            n174 = local write "Relay7"(w384) -> ()
          }
        }
      }
      frame True {
        w385 = FALSE ("Relay7")
        n175 = local write "Reclose Relay7?"(w385) -> ()
        n176 = local write "Relay7"(w385) -> ()
      }
    }
    n177 = case shown="True" w169 {
      frame False {
        "Trip Relay3" <- TRUE ("Reclose Relay1?")
      }
      frame True {
        n178 = local write "Reclose Relay3?"(TRUE ("Manual trip Relay1")) -> ()
        n179 = local write "Trip Relay3"(FALSE ("Manual trip Relay1")) -> ()
      }
    }
    n180 = case shown="True" w51 {
      tunnel: w52 -> [w379 _]
      frame False {
        n181 = case shown="True" w379 {
          selector: w379 -> [_ w380]
          frame False {
          }
          frame True {
            n182 = local write "Relay8"(w380) -> ()
          }
        }
      }
      frame True {
        w381 = FALSE ("Relay7")
        n183 = local write "Reclose Relay8?"(w381) -> ()
        n184 = local write "Relay8"(w381) -> ()
      }
    }
    n185 = feedback #17() -> (w367:bool)  [unwired: 1 in]
    n186 = feedback-in #17("Manual trip Relay1") -> ()
    n187 = feedback #18() -> (w239:bool)  [unwired: 1 in]
    n188 = feedback-in #18("Manual trip Relay4") -> ()
    n189 = feedback #19() -> (w130:bool)  [unwired: 1 in]
    n190 = feedback-in #19("Manual trip Relay5") -> ()
    n191 = feedback #20() -> (w84:bool)  [unwired: 1 in]
    n192 = feedback-in #20("Manual trip Relay6") -> ()
    n193 = feedback #21() -> (w40:bool)  [unwired: 1 in]
    n194 = feedback-in #21("Manual trip Relay8") -> ()
    n195 = feedback #22() -> (w81:bool)  [unwired: 1 in]
    n196 = feedback-in #22("Manual trip Relay7") -> ()
    n197 = feedback #23() -> (w297:bool)  [unwired: 1 in]
    n198 = feedback-in #23("Manual trip Relay2") -> ()
    n199 = feedback #24() -> (w294:bool)  [unwired: 1 in]
    n200 = feedback-in #24("Manual trip Relay3") -> ()
    n201 = local read "Trip Relay8"() -> (w36:bool)
    n202 = local read "Trip Relay2"() -> (w158:bool)
    n203 = local read "Trip Relay7"() -> (w34:bool)
    n204 = local read "Trip Relay5"() -> (w30:bool)
    n205 = local read "Trip Relay1"() -> (w156:bool)
    n206 = local read "Trip Relay3"() -> (w160:bool)
    n207 = local read "Trip Relay4"() -> (w162:bool)
    n208 = local read "Trip Relay6"() -> (w32:bool)
    n209 = Not Equal?(x="Manual trip Relay1", y=w367) -> (x != y?=w366:bool)
    n210 = Not Equal?(x="Manual trip Relay4", y=w239) -> (x != y?=w240:bool)
    n211 = Not Equal?(x="Manual trip Relay5", y=w130) -> (x != y?=w129:bool)
    n212 = Not Equal?(x="Manual trip Relay6", y=w84) -> (x != y?=w85:bool)
    n213 = Not Equal?(x="Manual trip Relay8", y=w40) -> (x != y?=w41:bool)
    n214 = Not Equal?(x="Manual trip Relay7", y=w81) -> (x != y?=w80:bool)
    n215 = Not Equal?(x="Manual trip Relay2", y=w297) -> (x != y?=w298:bool)
    n216 = Not Equal?(x="Manual trip Relay3", y=w294) -> (x != y?=w293:bool)
    n217 = And(x="Manual trip Relay1", y=w366) -> (x .and. y?=w364:bool)
    n218 = And(x="Manual trip Relay4", y=w240) -> (x .and. y?=w242:bool)
    n219 = And(x="Manual trip Relay5", y=w129) -> (x .and. y?=w127:bool)
    n220 = And(x="Manual trip Relay6", y=w85) -> (x .and. y?=w87:bool)
    n221 = And(x="Manual trip Relay8", y=w41) -> (x .and. y?=w43:bool)
    n222 = And(x="Manual trip Relay7", y=w80) -> (x .and. y?=w78:bool)
    n223 = And(x="Manual trip Relay2", y=w298) -> (x .and. y?=w300:bool)
    n224 = And(x="Manual trip Relay3", y=w293) -> (x .and. y?=w291:bool)
    n225 = Or(x=w127, y=w30) -> (x .or. y?=w31:bool)
    n226 = Or(x=w364, y=w156) -> (x .or. y?=w157:bool)
    n227 = Or(x=w78, y=w34) -> (x .or. y?=w35:bool)
    n228 = Or(x=w242, y=w162) -> (x .or. y?=w163:bool)
    n229 = Or(x=w87, y=w32) -> (x .or. y?=w33:bool)
    n230 = Or(x=w300, y=w158) -> (x .or. y?=w159:bool)
    n231 = Or(x=w291, y=w160) -> (x .or. y?=w161:bool)
    n232 = Or(x=w43, y=w36) -> (x .or. y?=w37:bool)
    n233 = case shown="True" w164 {
      frame False {
        "Trip Relay8" <- TRUE ("Manual trip Relay1")
      }
      frame True {
        n234 = local write "Reclose Relay8?"(TRUE ("Reclose Relay1?")) -> ()
        n235 = local write "Trip Relay8"(FALSE ("Reclose Relay1?")) -> ()
      }
    }
    n236 = case shown="True" w31 {
      frame False {
      }
      frame True {
        w394 = FALSE ("Relay7")
        n237 = local write "Reclose Relay5?"(w394) -> ()
        n238 = local write "Relay5"(w394) -> ()
      }
    }
    n239 = case shown="True" w168 {
      frame False {
        "Trip Relay4" <- TRUE ("Manual trip Relay1")
      }
      frame True {
        n240 = local write "Reclose Relay4?"(TRUE ("Reclose Relay1?")) -> ()
        n241 = local write "Trip Relay4"(FALSE ("Trip Relay4")) -> ()
      }
    }
    n242 = case shown="True" w157 {
      frame False {
      }
      frame True {
        w511 = FALSE ("Relay7")
        n243 = local write "Reclose Relay1?"(w511) -> ()
        n244 = local write "Relay1"(w511) -> ()
      }
    }
    n245 = case shown="True" w163 {
      frame False {
      }
      frame True {
        w425 = FALSE ("Relay7")
        n246 = local write "Reclose Relay4?"(w425) -> ()
        n247 = local write "Relay4"(w425) -> ()
      }
    }
    n248 = case shown="True" w33 {
      frame False {
      }
      frame True {
        w390 = FALSE ("Relay7")
        n249 = local write "Reclose Relay6?"(w390) -> ()
        n250 = local write "Relay6"(w390) -> ()
      }
    }
    n251 = case shown="True" w35 {
      frame False {
      }
      frame True {
        w386 = FALSE ("Relay7")
        n252 = local write "Reclose Relay7?"(w386) -> ()
        n253 = local write "Relay7"(w386) -> ()
      }
    }
    n254 = case shown="True" w161 {
      frame False {
      }
      frame True {
        w429 = FALSE ("Relay7")
        n255 = local write "Reclose Relay3?"(w429) -> ()
        n256 = local write "Relay3"(w429) -> ()
      }
    }
    n257 = case shown="True" w37 {
      frame False {
      }
      frame True {
        w382 = FALSE ("Relay7")
        n258 = local write "Reclose Relay8?"(w382) -> ()
        n259 = local write "Relay8"(w382) -> ()
      }
    }
    n260 = case shown="True" w159 {
      frame False {
      }
      frame True {
        w433 = FALSE ("Relay7")
        n261 = local write "Reclose Relay2?"(w433) -> ()
        n262 = local write "Relay2"(w433) -> ()
      }
    }
    n263 = Subtract(x=w150, y=w149) -> (x-y=w148:dbl)
    n264 = Build Array (concatenate)(w186, w185, w184, w183, w182, w181, w180, w179) -> (w187:dbl[])
    n265 = shared-variable "IntelliRupter\\IntelliRupter_data.lvlib\\Relay7_Ang_Diff"(w151) -> ()  [unwired: 1 in, 1 out]
    n266 = shared-variable "IntelliRupter\\IntelliRupter_data.lvlib\\Relay7_Freq_Diff"(w148) -> ()  [unwired: 1 in, 1 out]
    n267 = Tick Count (ms)() -> (millisecond timer value=w15:u32)
    n268 = shared-variable "IntelliRupter\\IntelliRupter_data.lvlib\\Relay_to_MGCC"(w187) -> ()  [unwired: 1 in, 1 out]
    n269 = shared-variable "IntelliRupter\\IntelliRupter_data.lvlib\\Relay7_Cmd"("Relay7") -> ()  [unwired: 1 in, 1 out]
    n270 = xnode "Read/Write Control"("FPGA VI Reference In"=w363, "Relay1"="Relay1", "Relay2"="Relay2", "Relay3"="Relay3", "Relay4"="Relay4", "Relay5"="Relay5", "Relay6"="Relay6", "Relay7"="Relay7", "Relay8"="Relay8", "Count(ticks)"="Count(ticks)") -> ("FPGA VI Reference Out"=w369:refnum<k20>, "error out"=w368:errorcluster)  [unwired: 1 in]
    n271 = feedback-in #25(w15) -> ()
    n272 = feedback #25() -> (w14:u32)  [unwired: 1 in]
    n273 = Subtract(x=w15, y=w14) -> (x-y=→"x-y":u32)
  }
  n274 = xnode "Close FPGA VI Reference"("FPGA VI Reference In"=w9, "error in"=w8) -> ()  [unwired: 1 out]
